vi "Autonomous.vi"() -> (1 "Boolean 2":bool, 2 "Boolean":bool, 3 "output cluster":T1)   [LabVIEW 2014]
panel:
  in  "stop":bool
  in  "Switch to Teleop":bool
  in  "Team Number":string
  in  "Comments":string
  in  "Did Your Robot Move a Crate\n into Auto Zone":string(combo)
  in  "Did Your Robot Move a Can\n into Auto Zone":string(combo)
  in  "Is Your Robot in Auto Zone":string(combo)
  in  "Position of Robot":string(combo)
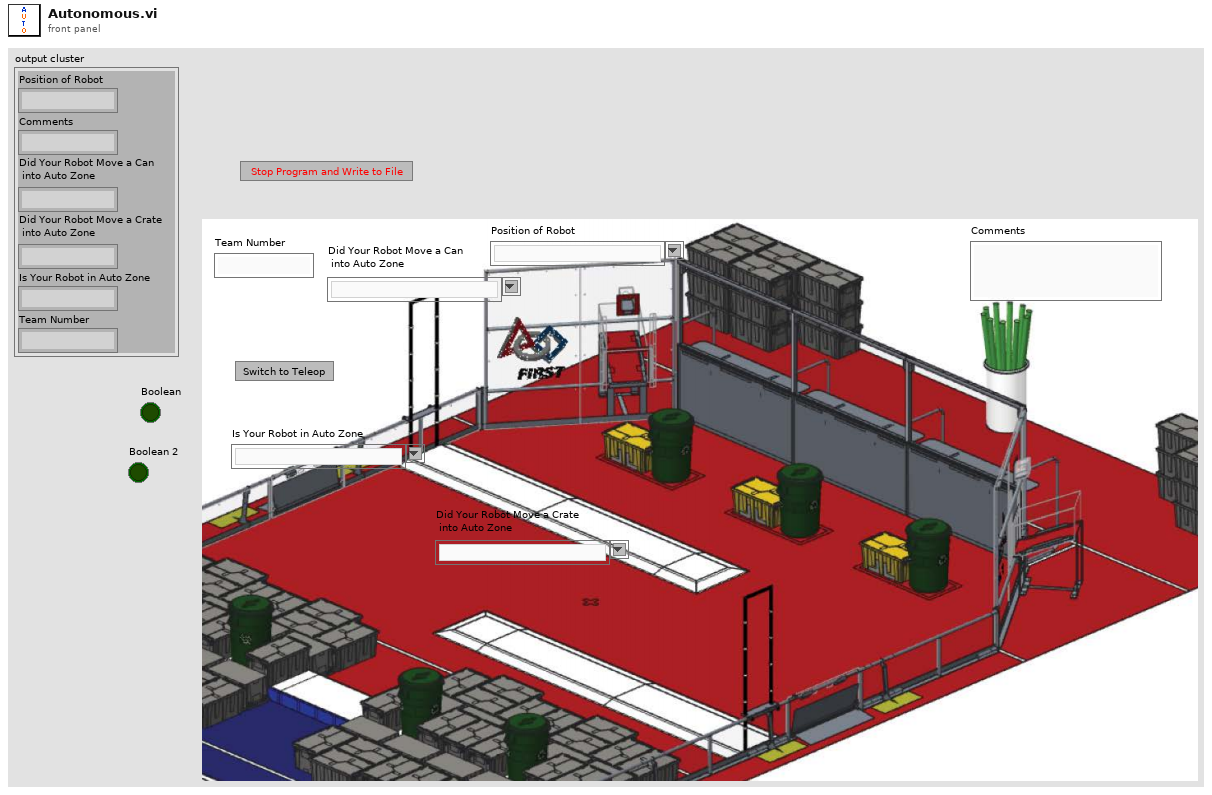
[diagram p1: front panel]
types:
  T1 = cluster{"Position of Robot":string, "Comments":string, "Did Your Robot Move a Can\n into Auto Zone":string, "Did Your Robot Move a Crate\n into Auto Zone ":string, "Is Your Robot in Auto Zone":string, "Team Number":string}
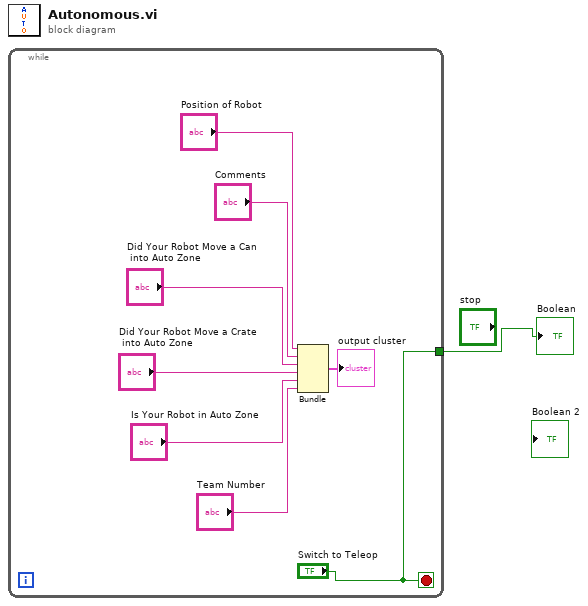
[diagram p0: block diagram]
diagram:
  n1 = while {
    tunnel: ["Switch to Teleop"] -> w1
    stop <- "Switch to Teleop" stop-if-true
    n2 = Bundle("Position of Robot"="Position of Robot", "Comments"="Comments", "Did Your Robot Move a Can\n into Auto Zone"="Did Your Robot Move a Can\n into Auto Zone", "Did Your Robot Move a Crate\n into Auto Zone"="Did Your Robot Move a Crate\n into Auto Zone", "Is Your Robot in Auto Zone"="Is Your Robot in Auto Zone", "Team Number"="Team Number") -> (→"output cluster":T1)  [unwired: 1 in]
  }
  "Boolean" <- w1
